vi "Drive Control.vi"(10 "Drive Powers":cluster{"Linear":dbl, "Turn":dbl}, 11 "Enum":enum16{"Run", "End", "Start"}(ring)) -> ()   [LabVIEW 2014]
uses:
  <vilib>/Rock Robotics/SystemInterfaces/DIO/FPGA_DIOPWMChannel.ctl
  <vilib>/Rock Robotics/WPI/MotorControl/WPI_MotorControlOpen Talon.vi
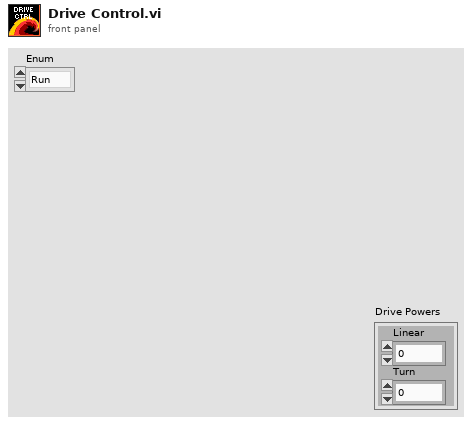
[diagram p1: front panel]
types:
  T1 = typedef "FPGA_DIOPWMChannel.ctl" = enum8{"PWM 0", "PWM 1", "PWM 2", "PWM 3", "PWM 4", "PWM 5", "PWM 6", "PWM 7", "PWM 8", "PWM 9", "PWM MXP 0", "PWM MXP 1", "PWM MXP 2", "PWM MXP 3", "PWM MXP 4", "PWM MXP 5", "PWM MXP 6", "PWM MXP 7", "PWM MXP 8", "PWM MXP 9", "Invalid"}
  T2 = typedef "WPI_MotorControlDeviceRef.ctl" = cluster{"DeviceStatus":errorcluster, "Type":T3, "PWM":cluster{"Controller":T4, "PWM Channel":T1, "DeadBand":T5}, "CAN":cluster{"Device Number":u8, "Control Mode":T6, "Semaphore":T7, "Max Vout":dbl, "TalonSRX Control Mode":T8}, "Invert":bool, "TransformRef":T9, "InvTransformRef":T9}
  T3 = typedef "WPI_MotorControlType.ctl" = enum16{"PWM", "CAN", "CANTalonSRX"}
  T4 = typedef "FPGA_TypedefDigitalModule.ctl" = enum16{"Controller 1"}
  T5 = typedef "WPI_PWMDeadband.ctl" = cluster{"Name":string, "maxPositivePwm":i32, "minPositivePwm":i32, "centerPwm":i32, "maxNegativePwm":i32, "minNegativePwm":i32, "angularRange":u16}
  T6 = typedef "WPI_CANJaguar_ControlMode.ctl" = enum8{"Percent VBus", "Current", "Speed", "Position", "Voltage"}
  T7 = typedef "Semaphore RefNum" = refnum<k1>
  T8 = typedef "WPI_CANTalonSRX_APIControlMode.ctl" = enum8{"Percent VBus", "Speed", "Position", "Slave", "Unchanged / Invalid"}
  T9 = typedef "WPI_PWMTransform_ConPane.ctl" = refnum<vi>
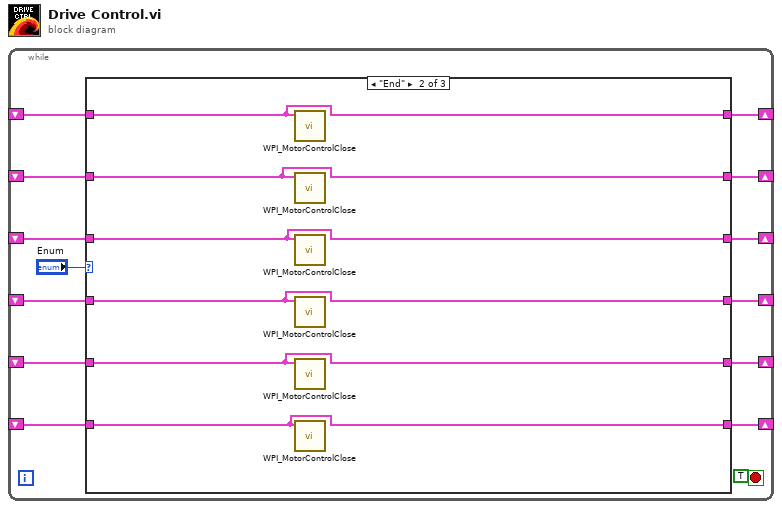
[diagram p0: block diagram]
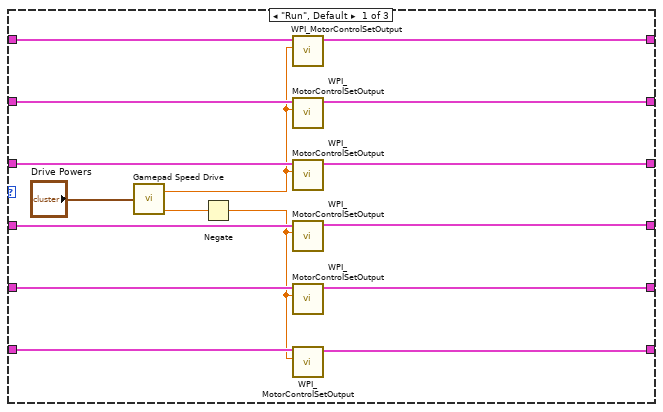
[diagram p2: hidden frame]
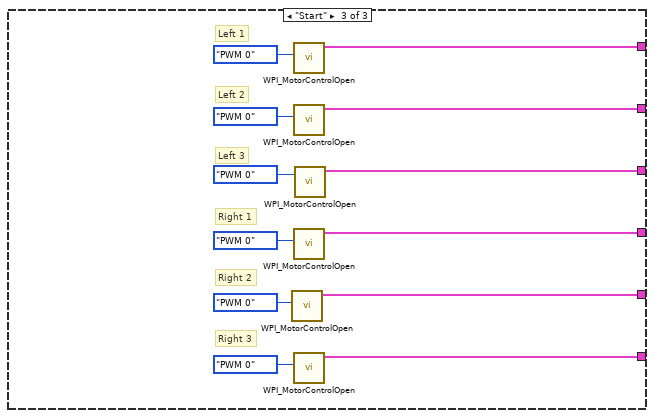
[diagram p3: hidden frame]
diagram:
  n1 = while {
    shift-right: [w14] -> _
    shift-left: _ -> [w1]
    shift-right: [w13] -> _
    shift-left: _ -> [w2]
    shift-right: [w12] -> _
    shift-left: _ -> [w6]
    shift-right: [w11] -> _
    shift-left: _ -> [w5]
    shift-right: [w10] -> _
    shift-left: _ -> [w4]
    shift-right: [w9] -> _
    shift-left: _ -> [w3]
    stop <- TRUE stop-if-true
    n2 = case shown="\"End\"" "Enum" {
      tunnel: [w20 w36 w48] -> w14
      tunnel: [w19 w35 w47] -> w13
      tunnel: [w18 w34 w46] -> w12
      tunnel: [w17 w33 w45] -> w11
      tunnel: [w16 w32 w44] -> w10
      tunnel: [w15 w31 w43] -> w9
      tunnel: w6 -> [w28 w34 _]
      tunnel: w5 -> [w27 w33 _]
      tunnel: w4 -> [w26 w32 _]
      tunnel: w3 -> [w25 w31 _]
      tunnel: w2 -> [w29 w35 _]
      tunnel: w1 -> [w30 w36 _]
      frame "Run", Default {
        n3 = call "Gamepad Speed Drive.vi"("Drive Powers"="Drive Powers") -> ("Left Output"=w23:dbl, "Right Output"=w22:dbl)  [unwired: 1 in]
        n4 = Negate(x=w22) -> (-x=w21:dbl)
        n5 = call <vilib>:"WPI_MotorControlSetOutput.vi"("Output"=w23, "MotorControlDevRef"=w30) -> ("MotorControlDevRef"=w20:T2)  [unwired: 7 in, 2 out]
        n6 = call <vilib>:"WPI_MotorControlSetOutput.vi"("Output"=w23, "MotorControlDevRef"=w29) -> ("MotorControlDevRef"=w19:T2)  [unwired: 7 in, 2 out]
        n7 = call <vilib>:"WPI_MotorControlSetOutput.vi"("Output"=w23, "MotorControlDevRef"=w28) -> ("MotorControlDevRef"=w18:T2)  [unwired: 7 in, 2 out]
        n8 = call <vilib>:"WPI_MotorControlSetOutput.vi"("Output"=w21, "MotorControlDevRef"=w27) -> ("MotorControlDevRef"=w17:T2)  [unwired: 7 in, 2 out]
        n9 = call <vilib>:"WPI_MotorControlSetOutput.vi"("Output"=w21, "MotorControlDevRef"=w26) -> ("MotorControlDevRef"=w16:T2)  [unwired: 7 in, 2 out]
        n10 = call <vilib>:"WPI_MotorControlSetOutput.vi"("Output"=w21, "MotorControlDevRef"=w25) -> ("MotorControlDevRef"=w15:T2)  [unwired: 7 in, 2 out]
      }
      frame "End" {
        n11 = call <vilib>:"WPI_MotorControlClose.vi"("MotorControlDevRef"=w36) -> ()  [unwired: 10 in, 1 out]
        n12 = call <vilib>:"WPI_MotorControlClose.vi"("MotorControlDevRef"=w35) -> ()  [unwired: 10 in, 1 out]
        n13 = call <vilib>:"WPI_MotorControlClose.vi"("MotorControlDevRef"=w34) -> ()  [unwired: 10 in, 1 out]
        n14 = call <vilib>:"WPI_MotorControlClose.vi"("MotorControlDevRef"=w33) -> ()  [unwired: 10 in, 1 out]
        n15 = call <vilib>:"WPI_MotorControlClose.vi"("MotorControlDevRef"=w32) -> ()  [unwired: 10 in, 1 out]
        n16 = call <vilib>:"WPI_MotorControlClose.vi"("MotorControlDevRef"=w31) -> ()  [unwired: 10 in, 1 out]
      }
      frame "Start" {
        # "Right 3"
        # "Right 2"
        # "Right 1"
        # "Left 3"
        # "Left 2"
        # "Left 1"
        n17 = call-poly <vilib>:"WPI_MotorControlOpen.vi"("PWM Channel"=FPGA_DIOPWMChannel."PWM 0") -> ("MotorControlDeviceRef"=w44:T2)  [unwired: 9 in, 1 out]
        n18 = call-poly <vilib>:"WPI_MotorControlOpen.vi"("PWM Channel"=FPGA_DIOPWMChannel."PWM 0") -> ("MotorControlDeviceRef"=w48:T2)  [unwired: 9 in, 1 out]
        n19 = call-poly <vilib>:"WPI_MotorControlOpen.vi"("PWM Channel"=FPGA_DIOPWMChannel."PWM 0") -> ("MotorControlDeviceRef"=w47:T2)  [unwired: 9 in, 1 out]
        n20 = call-poly <vilib>:"WPI_MotorControlOpen.vi"("PWM Channel"=FPGA_DIOPWMChannel."PWM 0") -> ("MotorControlDeviceRef"=w45:T2)  [unwired: 9 in, 1 out]
        n21 = call-poly <vilib>:"WPI_MotorControlOpen.vi"("PWM Channel"=FPGA_DIOPWMChannel."PWM 0") -> ("MotorControlDeviceRef"=w43:T2)  [unwired: 9 in, 1 out]
        n22 = call-poly <vilib>:"WPI_MotorControlOpen.vi"("PWM Channel"=FPGA_DIOPWMChannel."PWM 0") -> ("MotorControlDeviceRef"=w46:T2)  [unwired: 9 in, 1 out]
      }
    }
  }
